vi "SW_Set_Adv_Stimulus_interface.vi"(0 "Zone-based stimulus presents":T1(array[cluster])=[{"Event type"=0, "Time, s"=0.0, "Stimulus, s"=0.0, "Set/Clear"=FALSE, "TTL out"=1, "Stim. has been set"=FALSE}, {"Event type"=0, "Time, s"=0.0, "Stimulus, s"=0.0, "Set/Clear"=FALSE, "TTL out"=1, "Stim. has been set"=FALSE}, {"Event type"=0, "Time, s"=0.0, "Stimulus, s"=0.0, "Set/Clear"=FALSE, "TTL out"=1, "Stim. has been set"=FALSE}, {"Event type"=0, "Time, s"=0.0, "Stimulus, s"=0.0, "Set/Clear"=FALSE, "TTL out"=1, "Stim. has been set"=FALSE}, {"Event type"=0, "Time, s"=0.0, "Stimulus, s"=0.0, "Set/Clear"=FALSE, "TTL out"=1, "Stim. has been set"=FALSE}, {"Event type"=0, "Time, s"=0.0, "Stimulus, s"=0.0, "Set/Clear"=FALSE, "TTL out"=1, "Stim. has been set"=FALSE}, {"Event type"=0, "Time, s"=0.0, "Stimulus, s"=0.0, "Set/Clear"=FALSE, "TTL out"=1, "Stim. has been set"=FALSE}, {"Event type"=0, "Time, s"=0.0, "Stimulus, s"=0.0, "Set/Clear"=FALSE, "TTL out"=1, "Stim. has been set"=FALSE}, {"Event type"=0, "Time, s"=0.0, "Stimulus, s"=0.0, "Set/Clear"=FALSE, "TTL out"=1, "Stim. has been set"=FALSE}, {"Event type"=0, "Time, s"=3.0, "Stimulus, s"=0.3, "Set/Clear"=TRUE, "TTL out"=3, "Stim. has been set"=TRUE}, {"Event type"=0, "Time, s"=0.0, "Stimulus, s"=0.0, "Set/Clear"=FALSE, "TTL out"=1, "Stim. has been set"=FALSE}, {"Event type"=0, "Time, s"=5.0, "Stimulus, s"=1.0, "Set/Clear"=TRUE, "TTL out"=1, "Stim. has been set"=TRUE}, {"Event type"=0, "Time, s"=2.0, "Stimulus, s"=1.0, "Set/Clear"=TRUE, "TTL out"=2, "Stim. has been set"=TRUE}, {"Event type"=0, "Time, s"=0.0, "Stimulus, s"=0.0, "Set/Clear"=FALSE, "TTL out"=1, "Stim. has been set"=FALSE}] {"Event type" items=["Time spent in zone", "Future options"]; "TTL out" items=["1"=1, "2"=2, "1 + 2"=3]}, 1 "Total amount of segments":u32=7, 7 "Run time, s":dbl, 9 "Run time stim, s":dbl, 11 "Run time pause, s":dbl, 12 "Run time threshold, s":dbl, 13 "Speed detection threshold, mm/s":dbl=8.0) -> (3 "Modified Zone-based stimulus presents":T1(array[cluster])=[{"Event type"=0, "Time, s"=0.0, "Stimulus, s"=0.0, "Set/Clear"=FALSE, "TTL out"=1, "Stim. has been set"=FALSE}, {"Event type"=0, "Time, s"=0.0, "Stimulus, s"=0.0, "Set/Clear"=FALSE, "TTL out"=1, "Stim. has been set"=FALSE}, {"Event type"=0, "Time, s"=0.0, "Stimulus, s"=0.0, "Set/Clear"=FALSE, "TTL out"=1, "Stim. has been set"=FALSE}, {"Event type"=0, "Time, s"=0.0, "Stimulus, s"=0.0, "Set/Clear"=FALSE, "TTL out"=1, "Stim. has been set"=FALSE}, {"Event type"=0, "Time, s"=0.0, "Stimulus, s"=0.0, "Set/Clear"=FALSE, "TTL out"=1, "Stim. has been set"=FALSE}, {"Event type"=0, "Time, s"=0.0, "Stimulus, s"=0.0, "Set/Clear"=FALSE, "TTL out"=1, "Stim. has been set"=FALSE}, {"Event type"=0, "Time, s"=0.0, "Stimulus, s"=0.0, "Set/Clear"=FALSE, "TTL out"=1, "Stim. has been set"=FALSE}, {"Event type"=0, "Time, s"=0.0, "Stimulus, s"=0.0, "Set/Clear"=FALSE, "TTL out"=1, "Stim. has been set"=FALSE}, {"Event type"=0, "Time, s"=0.0, "Stimulus, s"=0.0, "Set/Clear"=FALSE, "TTL out"=1, "Stim. has been set"=FALSE}, {"Event type"=0, "Time, s"=3.0, "Stimulus, s"=0.3, "Set/Clear"=TRUE, "TTL out"=3, "Stim. has been set"=TRUE}, {"Event type"=0, "Time, s"=0.0, "Stimulus, s"=0.0, "Set/Clear"=FALSE, "TTL out"=1, "Stim. has been set"=FALSE}, {"Event type"=0, "Time, s"=5.0, "Stimulus, s"=1.0, "Set/Clear"=TRUE, "TTL out"=1, "Stim. has been set"=TRUE}, {"Event type"=0, "Time, s"=2.0, "Stimulus, s"=1.0, "Set/Clear"=TRUE, "TTL out"=2, "Stim. has been set"=TRUE}, {"Event type"=0, "Time, s"=0.0, "Stimulus, s"=0.0, "Set/Clear"=FALSE, "TTL out"=1, "Stim. has been set"=FALSE}] {"Event type" items=["Time spent in zone", "Future options"]; "TTL out" items=["1"=1, "2"=2, "1 + 2"=3]}, 4 "Out Run time, s":dbl, 6 "Out Run time stim, s":dbl, 8 "Out Run time pause, s":dbl, 10 "Out Run time threshold, s":dbl, 15 "Out Speed detection threshold, mm/s":dbl)   [LabVIEW 2016]
uses:
  <vilib>/Utility/miscctls.llb/LVPositionTypeDef.ctl
panel:
  in  "Parameter 5A":dbl=50.0 caption="Speed thresh., mm/s" min=0.0 max=1000.0 step=0.25 format="%.2g"
  out "NewVal":T1(array[cluster])
  out "OldVal":T1(array[cluster])
  in  "Update Zones":bool=TRUE
  in  "Parameter 4A":dbl=50.0 caption="Run time thr., s" min=0.0 max=1000.0 step=0.25 format="%.2g"
  in  "Parameter 3B":dbl=50.0 caption="Time, s" min=0.0 max=1000.0 step=0.25 format="%.2g"
  in  "Parameter 1B":u16(ring) caption="Zone #" items=["Zone 01", "Zone 02", "Zone 03", "Zone 04", "Zone 05", "Zone 06", "Zone 07", "Zone 08", "Zone 09", "Zone 10", "Zone 11", "Zone 12"]
  in  "Parameter 2B":u16(ring) caption="Event type" items=["Time spent in zone", "Future options"]
  in  "Parameter 5B":u16(ring) caption="TTL out" items=["1"=1, "2"=2, "1 + 2"=3]
  out "Navigate Tree:Get Path":string[](array[string])
  in  "Remove Button":bool=TRUE
  in  "Add Button":bool=TRUE
  in  "Modify Button":bool=TRUE
  in  "Reset settings":bool
  in  "Exit":bool
  in  "Save Settings":bool
  in  "Parameter 4B":dbl=50.0 caption="Stimulus, s" min=0.0 max=1000.0 step=0.25 format="%.2g"
  in  "Parameter 3A":dbl=50.0 caption="Stimulus, s" min=0.0 max=1000.0 step=0.25 format="%.2g"
  in  "Parameter 2A":dbl=50.0 caption="Pause, s" min=0.0 max=1000.0 step=0.25 format="%.2f"
  in  "Parameter 1A":dbl=50.0 caption="Runnig, s" min=0.0 max=1000.0 step=0.25 format="%.2g"
  in  "TTL firing conditions":string(tree)
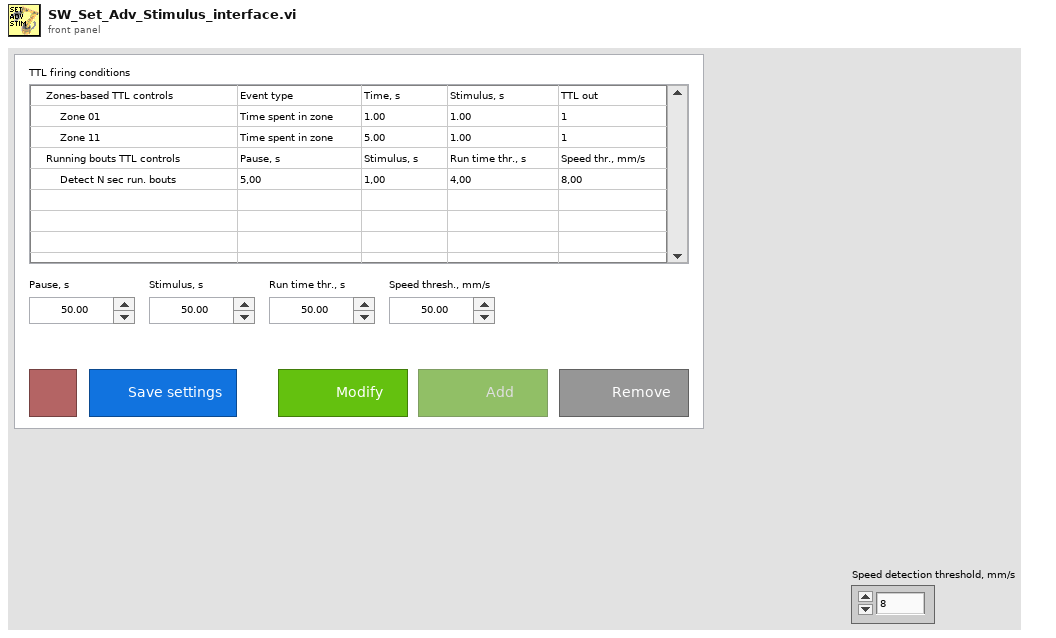
[diagram p1: front panel]
types:
  T1 = cluster{"Event type":u16, "Time, s":sgl, "Stimulus, s":sgl, "Set/Clear":bool, "TTL out":u16, "Stim. has been set":bool}[]
  T2 = typedef "LVPositionTypeDef.ctl" = cluster{"Left":i32, "Top":i32}
  T3 = typedef "LVStringsAndValuesArrayTypeDef_U16.ctl" = cluster{"String":string, "Value":u16}[]
  T4 = enum8{"Enabled", "Disabled", "Disabled and Grayed Out"}
  T5 = cluster{"Event type":u16, "Time, s":sgl, "Stimulus, s":sgl, "Set/Clear":bool, "TTL out":u16, "Stim. has been set":bool}
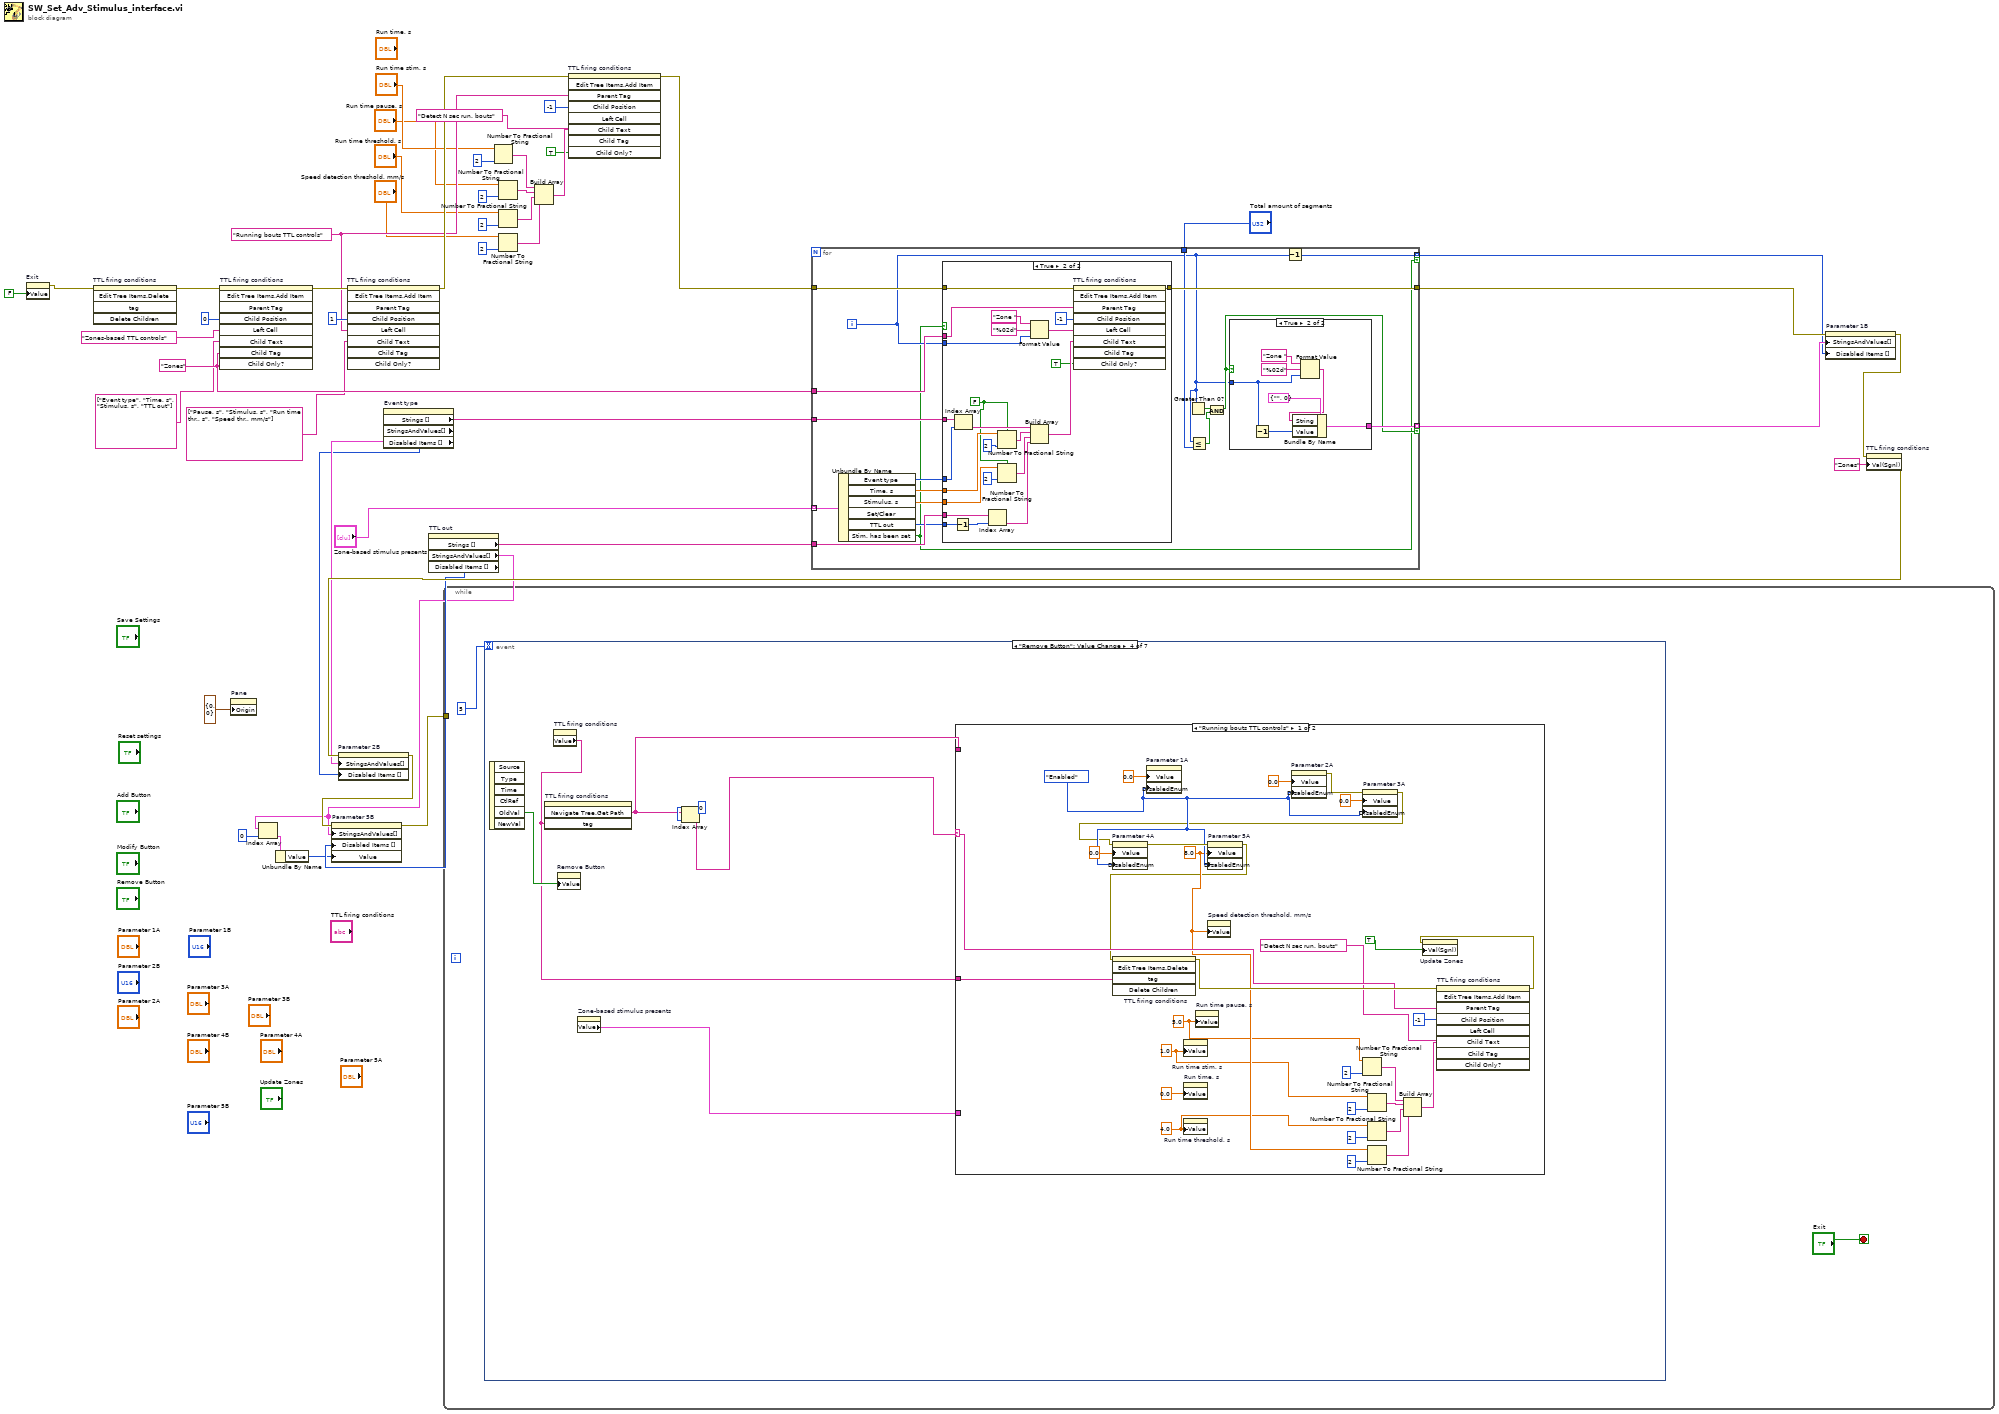
[diagram p0: block diagram]
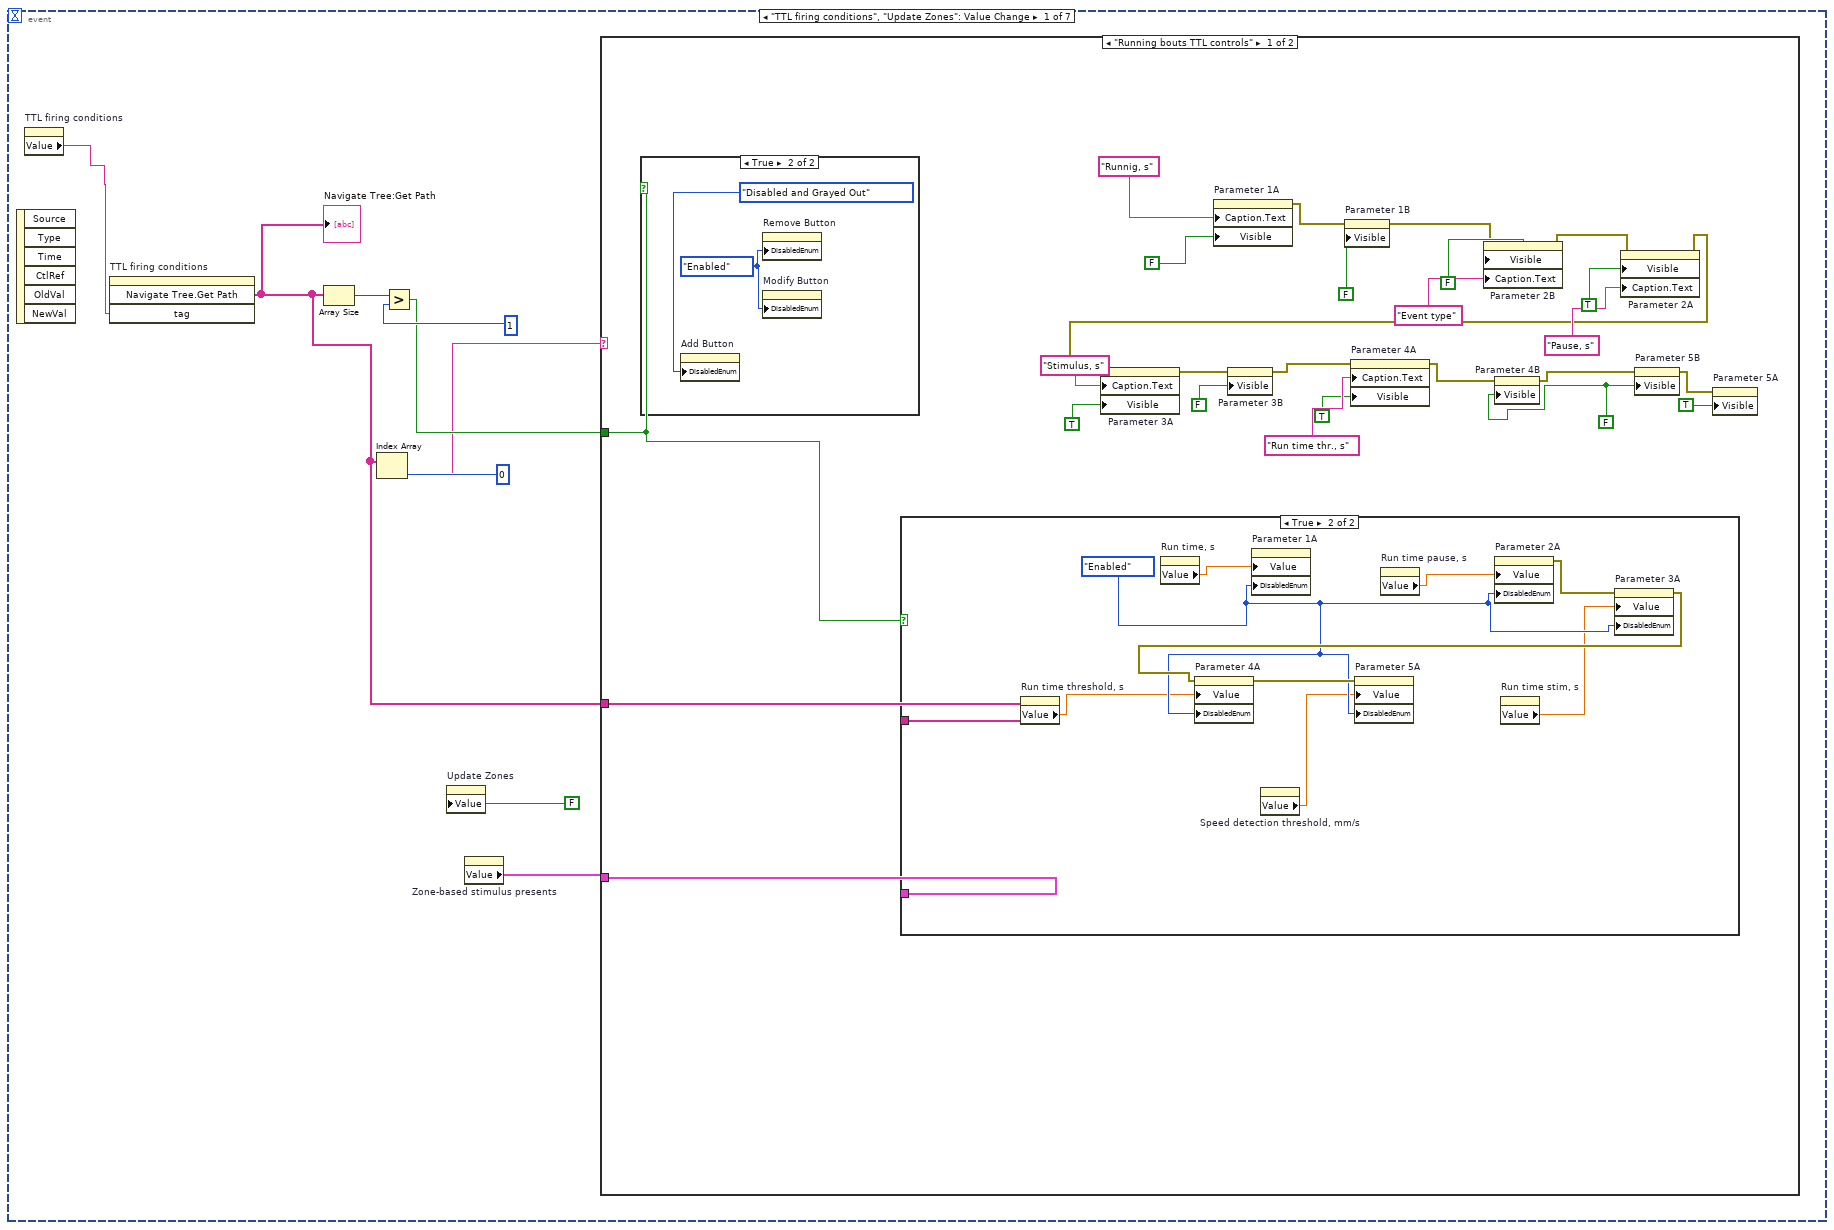
[diagram p2: hidden frame]
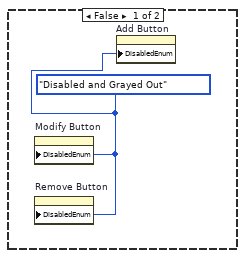
[diagram p3: hidden frame]
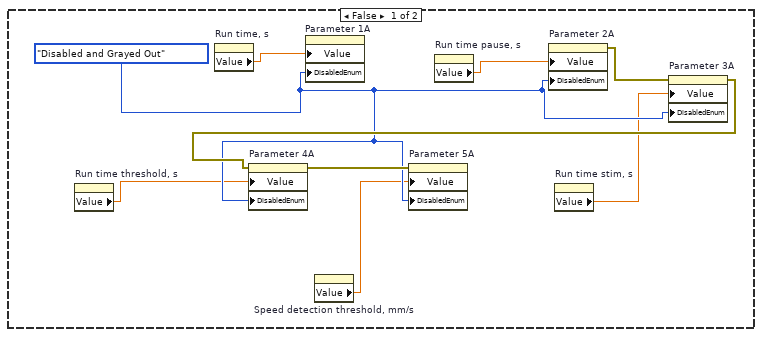
[diagram p4: hidden frame]
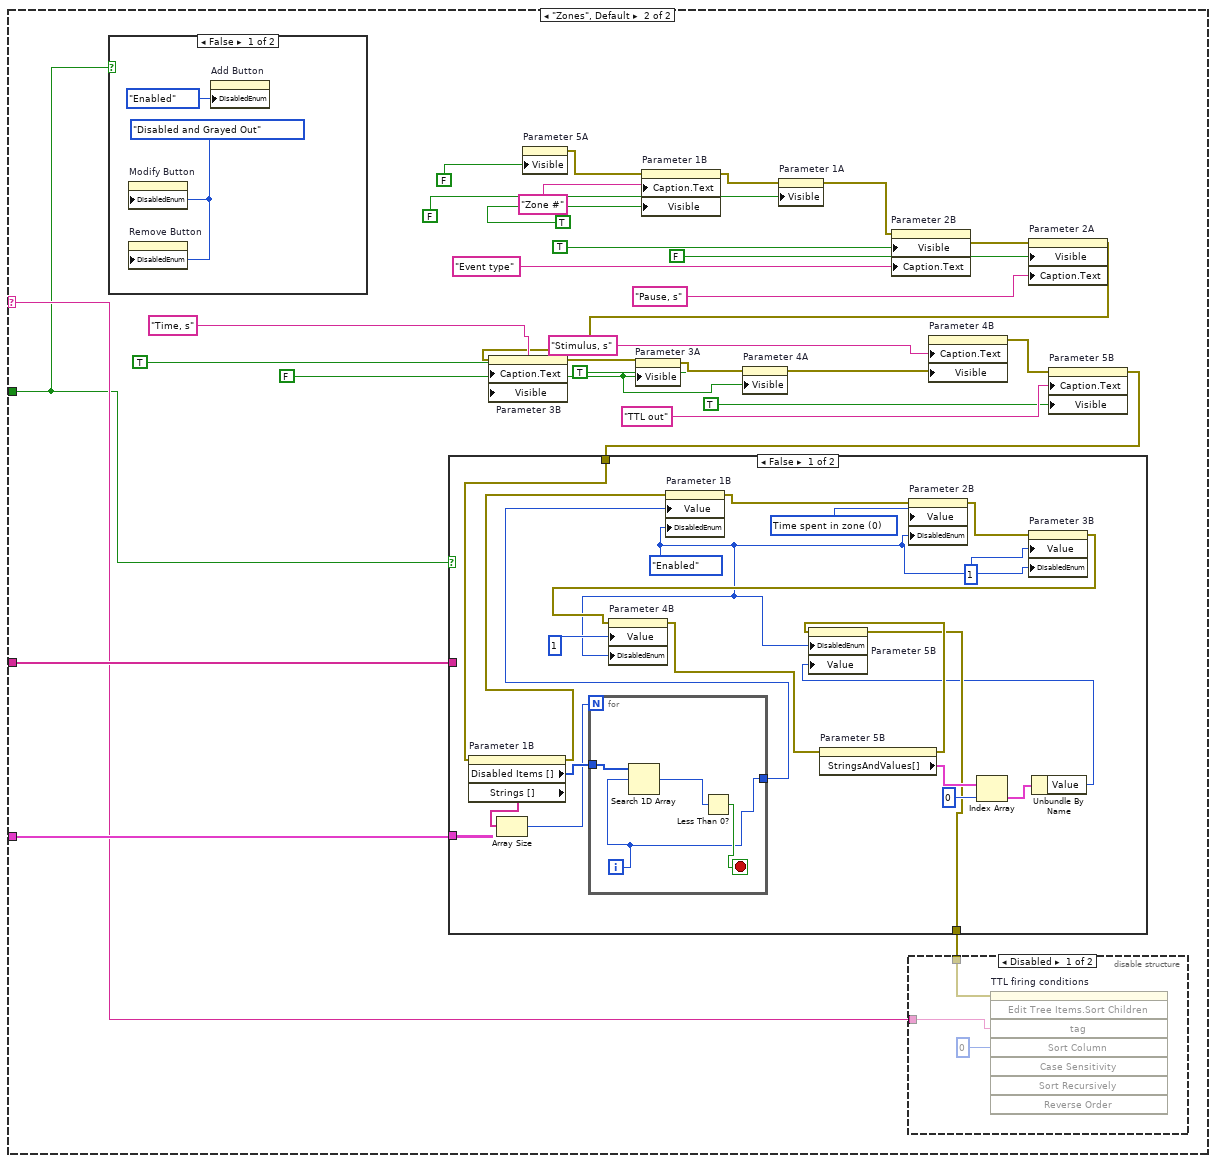
[diagram p5: hidden frame]
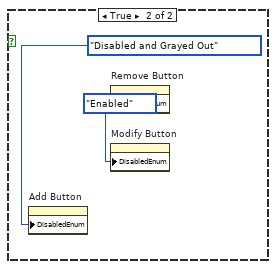
[diagram p6: hidden frame]
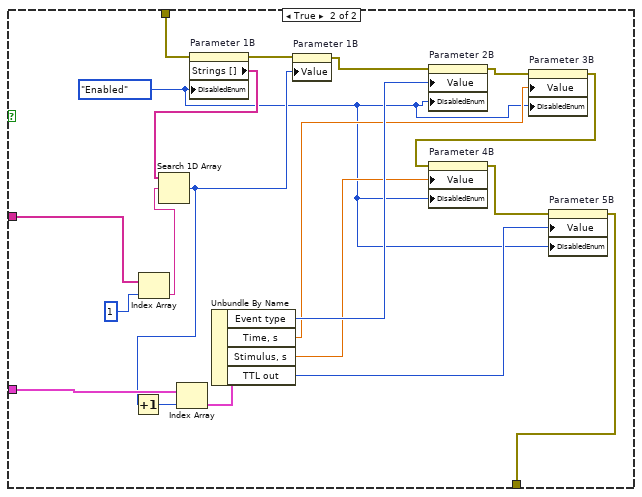
[diagram p8: hidden frame]
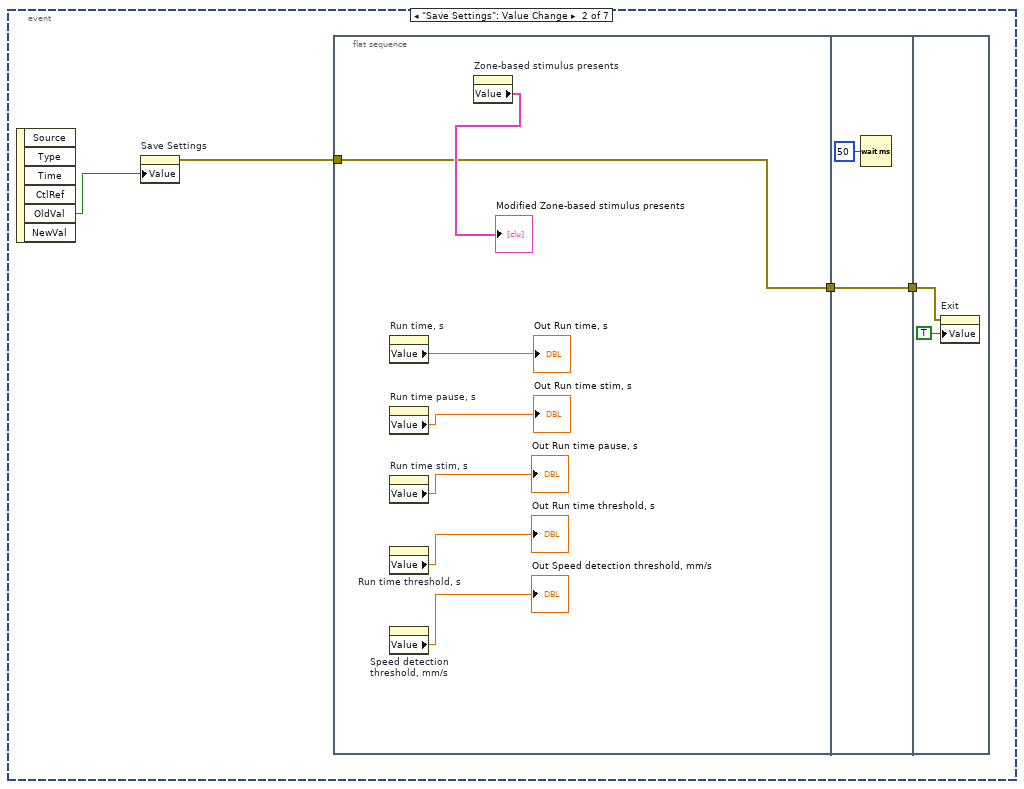
[diagram p9: hidden frame]
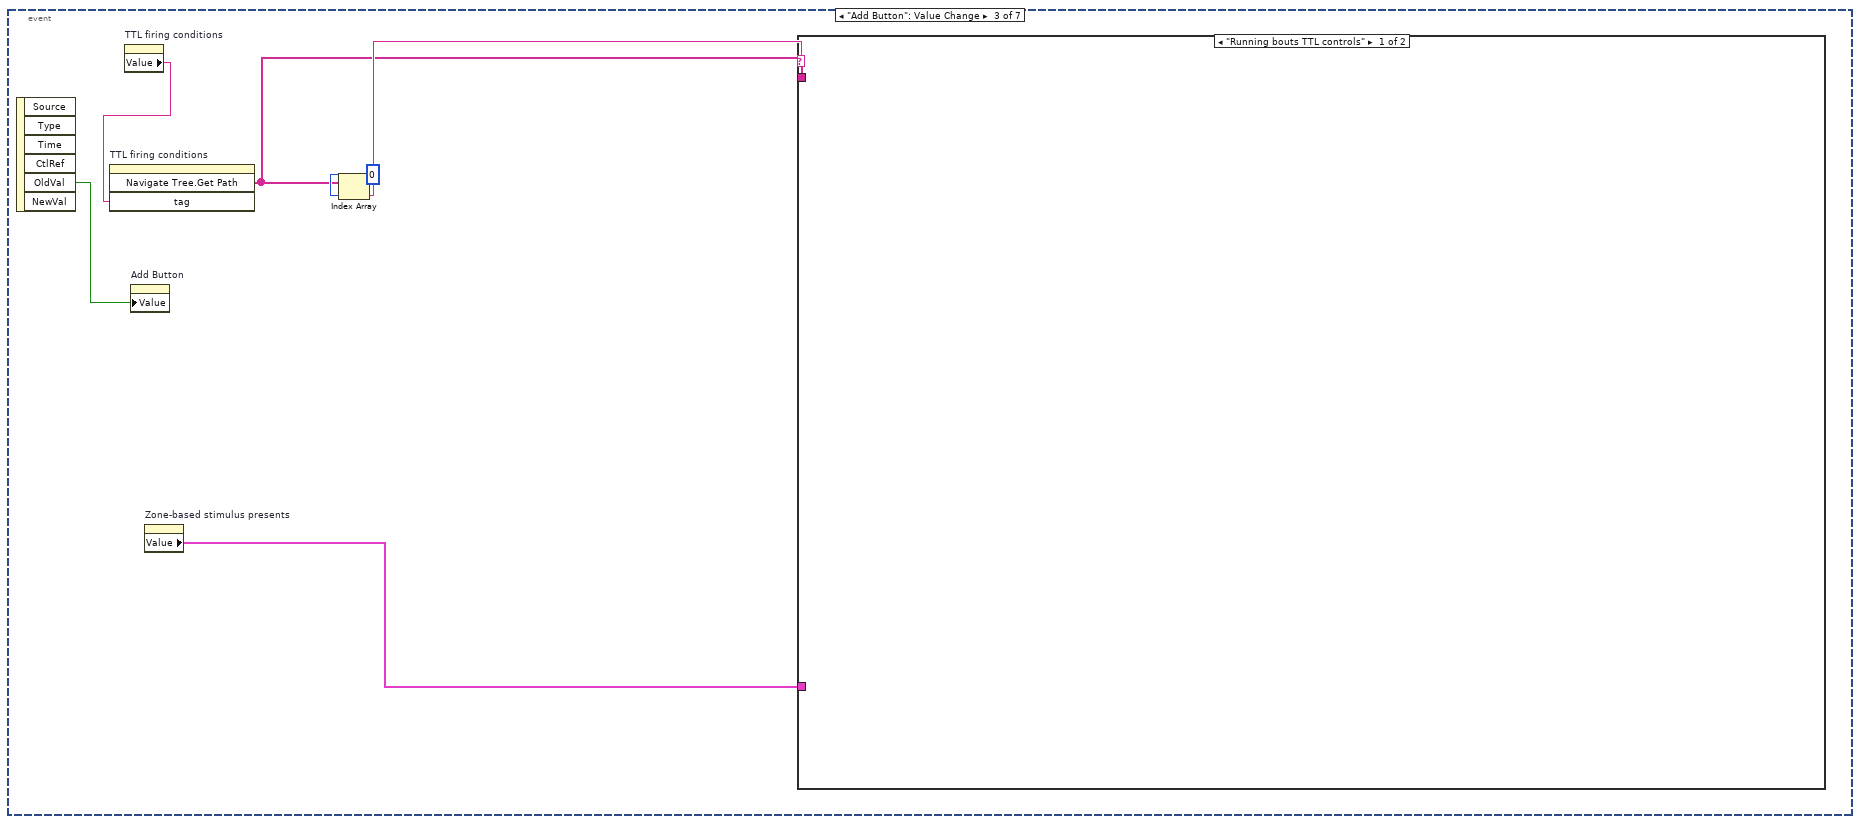
[diagram p10: hidden frame]
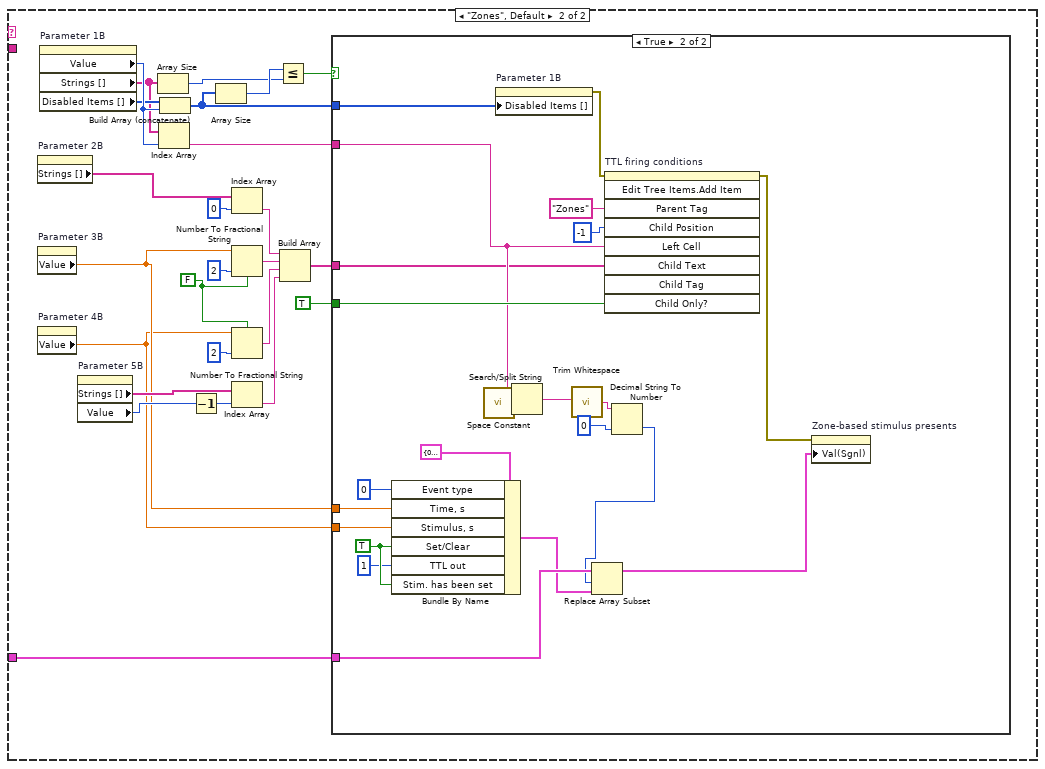
[diagram p11: hidden frame]
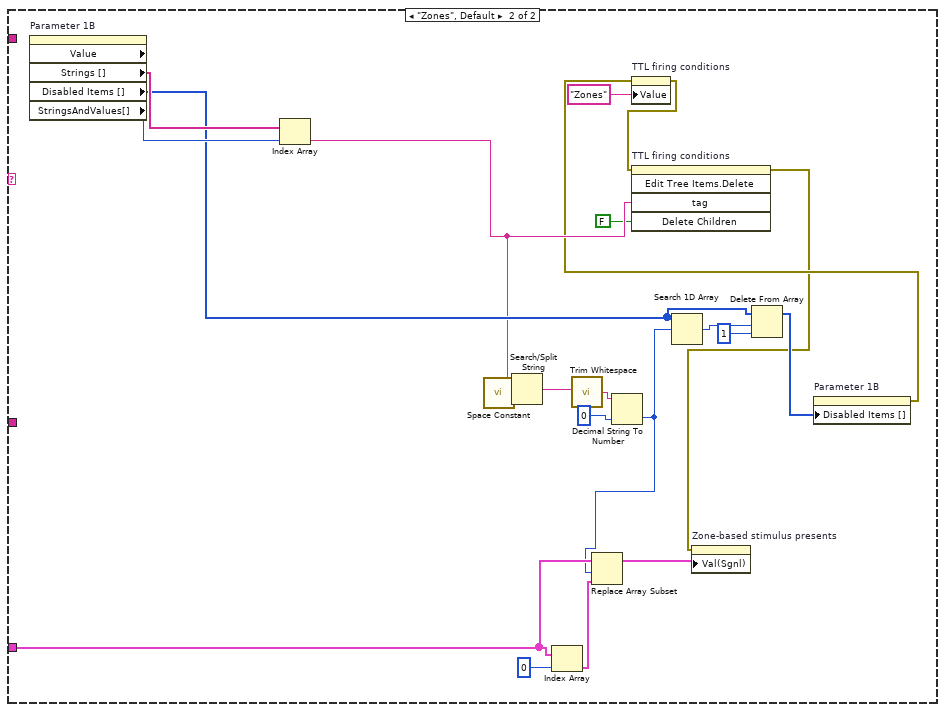
[diagram p13: hidden frame]
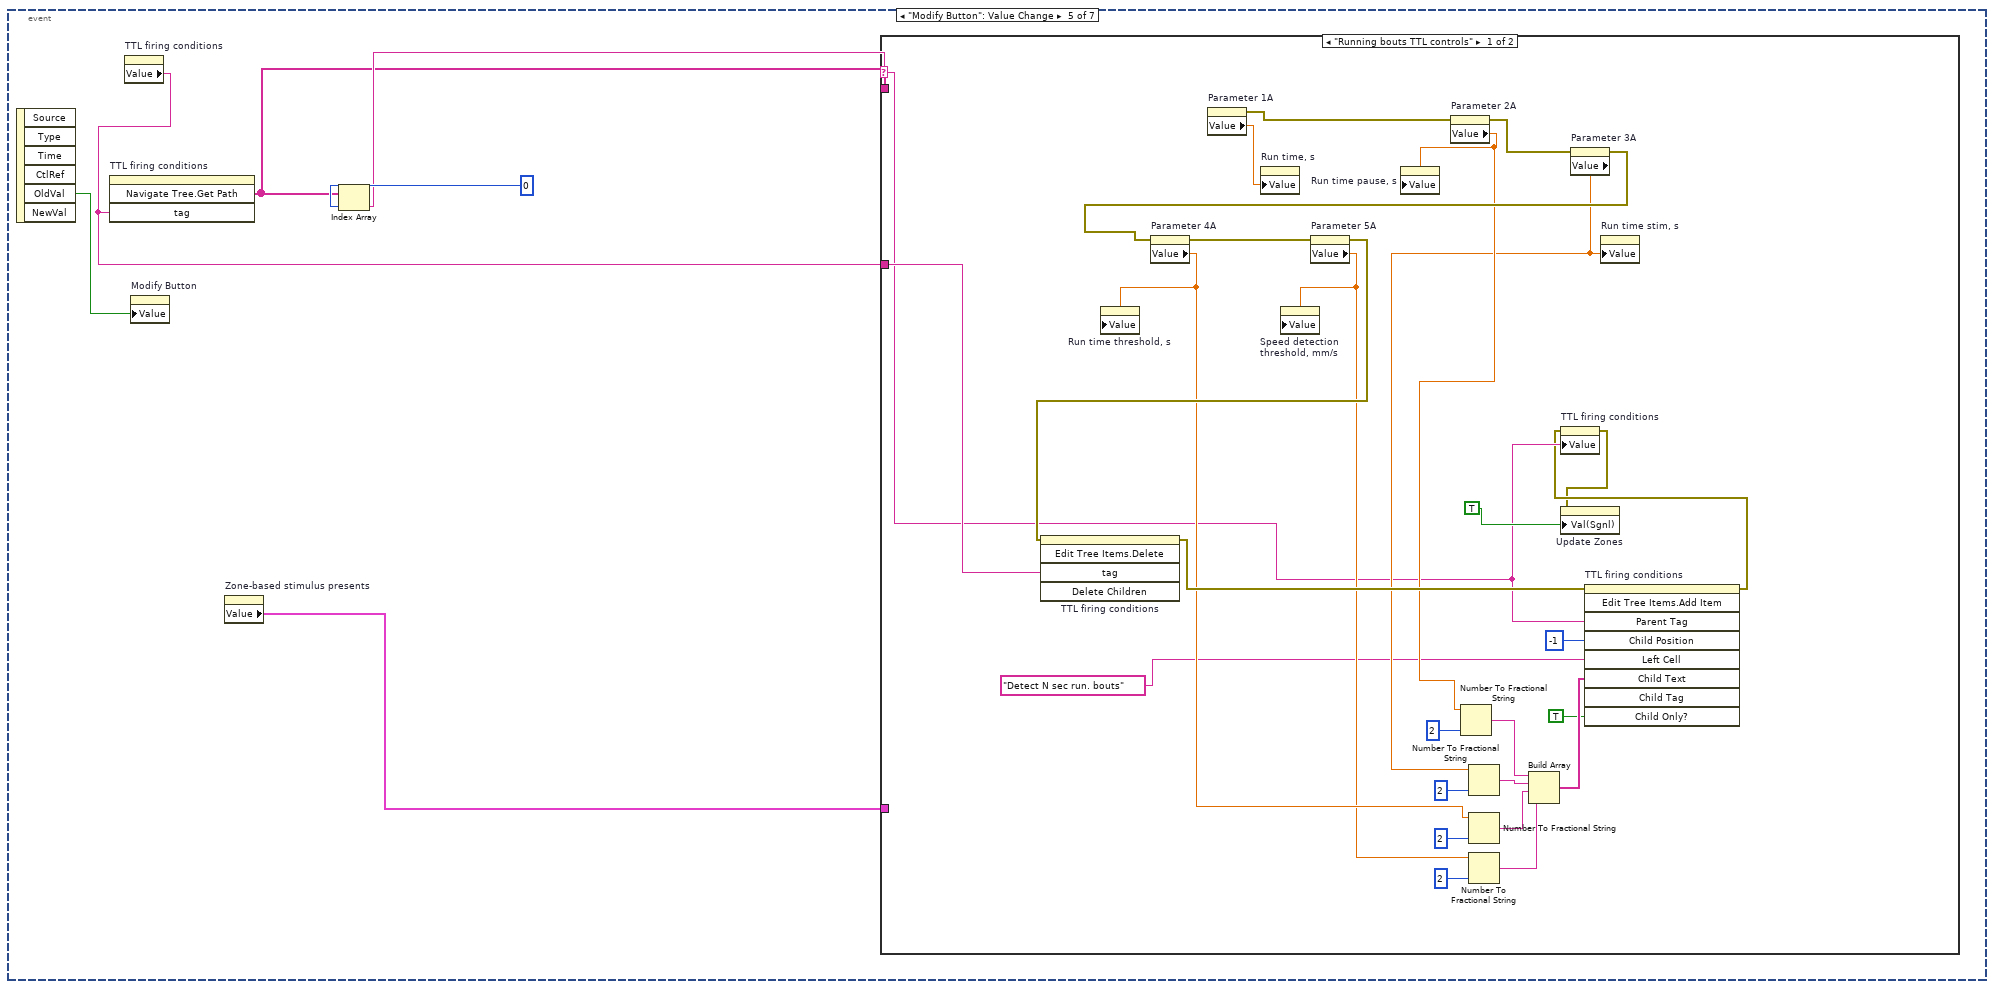
[diagram p14: hidden frame]
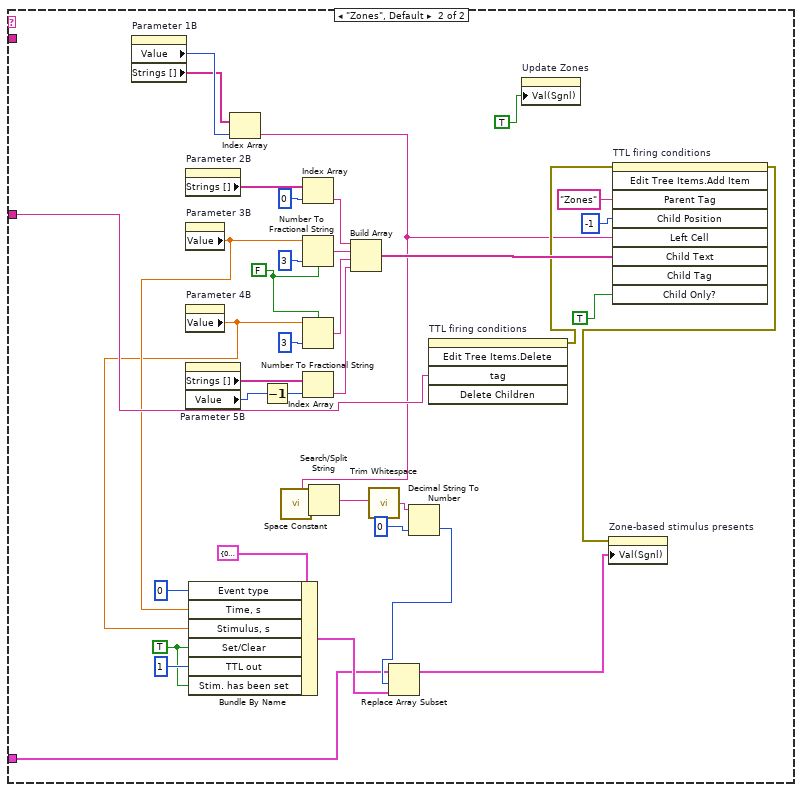
[diagram p15: hidden frame]
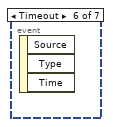
[diagram p16: hidden frame]
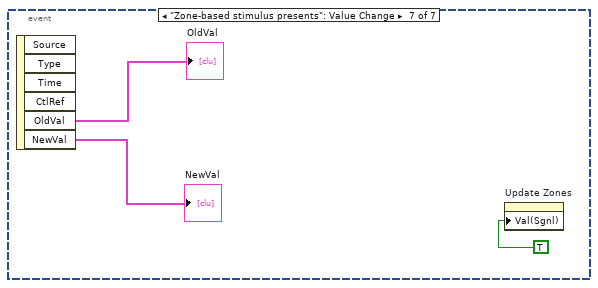
[diagram p17: hidden frame]
diagram:
  w19 = "Running bouts TTL controls" ("Parent Tag")
  w47 = "Zones" ("Child Tag")
  n1 = property on="Exit" class="Bool (strict)"("Value"=FALSE ("Exit")) -> (error out=w3:errorcluster)  [unwired: 2 in, 1 out]
  n2 = invoke on="TTL firing conditions" class="Tree (strict)" method="Edit Tree Items.Delete"(error in=w3) -> (error out=w48:errorcluster)  [unwired: 4 in, 4 out]
  n3 = invoke on="TTL firing conditions" class="Tree (strict)" method="Edit Tree Items.Add Item"(error in=w48, "Child Position"=0, "Left Cell"="Zones-based TTL controls" ("Parent Tag"), "Child Text"=string[] ["Event type", "Time, s", "Stimulus, s", "TTL out"], "Child Tag"=w47) -> (error out=w44:errorcluster)  [unwired: 4 in, 8 out]
  n4 = property on="Pane" class="Pane"("Origin"=T2 {"Left"=0, "Top"=0} ("Position")) -> ()  [unwired: 2 in, 2 out]
  n5 = invoke on="TTL firing conditions" class="Tree (strict)" method="Edit Tree Items.Add Item"(error in=w44, "Child Position"=1, "Left Cell"=w19, "Child Text"=string[] ["Pause, s", "Stimulus, s", "Run time thr., s", "Speed thr., mm/s"]) -> (error out=w21:errorcluster)  [unwired: 5 in, 8 out]
  n6 = property on="Event type" class="Ring (strict)"() -> ("Strings []"=w37:string[], "StringsAndValues[]"=w36:T3, "Disabled Items []"=w35:i32[])  [unwired: 2 in, 2 out]
  n7 = property on="TTL out" class="Ring (strict)"() -> ("Strings []"=w45:string[], "StringsAndValues[]"=w31:T3, "Disabled Items []"=w32:i32[])  [unwired: 2 in, 2 out]
  n8 = Index Array(array=w31, index=0) -> (element=w29:cluster{"String":string, "Value":u16})
  n9 = Unbundle By Name(w29) -> ("Value"=w28:u16)
  n10 = Number To Fractional String(number="Run time stim, s", precision (6)=i16 2) -> (F-format string=w9:string)  [unwired: 2 in]
  n11 = Number To Fractional String(number="Run time pause, s", precision (6)=i16 2) -> (F-format string=w8:string)  [unwired: 2 in]
  n12 = Number To Fractional String(number="Run time threshold, s", precision (6)=i16 2) -> (F-format string=w7:string)  [unwired: 2 in]
  n13 = Number To Fractional String(number="Speed detection threshold, mm/s", precision (6)=i16 2) -> (F-format string=w6:string)  [unwired: 2 in]
  n14 = Build Array(w9, w8, w7, w6) -> (w5:string[])
  n15 = invoke on="TTL firing conditions" class="Tree (strict)" method="Edit Tree Items.Add Item"(error in=w21, "Parent Tag"=w19, "Child Position"=-1, "Left Cell"="Detect N sec run. bouts" ("Left Cell String"), "Child Text"=w5, "Child Only?"=TRUE) -> (error out=w20:errorcluster)  [unwired: 3 in, 8 out]
  n16 = for {
    tunnel: "Zone-based stimulus presents" -> [w67] mode=indexing
    tunnel: w20 -> [w66]
    tunnel: w47 -> [w65]
    tunnel: w37 -> [w63]
    tunnel: w45 -> [w60]
    tunnel: [w58] -> w27
    tunnel: [w57] -> w26 mode=indexing if=w55
    tunnel: "Total amount of segments" -> [w56]
    tunnel: [w50] -> w24 mode=indexing if=w51
    i -> [w52]
    n17 = Unbundle By Name(w67) -> ("Event type"=w62:u16, "Time, s"=w64:sgl, "Stimulus, s"=w61:sgl, "TTL out"=w59:u16, "Stim. has been set"=w51:bool)  [unwired: 1 out]
    n18 = case shown="True" w51 {
      tunnel: w66 -> [_ w98]
      tunnel: w65 -> [_ w97]
      tunnel: w52 -> [_ w91]
      tunnel: w64 -> [_ w92]
      tunnel: w63 -> [_ w90]
      tunnel: w62 -> [_ w86]
      tunnel: w61 -> [_ w85]
      tunnel: w60 -> [_ w81]
      tunnel: w59 -> [_ w80]
      tunnel: [_ w76] -> w58
      frame False {
      }
      frame True {
        w75 = FALSE ("use system decimal point (T)")
        n19 = Decrement(x=w80) -> (x-1=w78:u16)
        n20 = Index Array(array=w90, index=w86) -> (element=w89:string)
        n21 = Index Array(array=w81, index=w78) -> (element=w79:string)
        n22 = Number To Fractional String(use system decimal point (T)=w75, number=w92, precision (6)=i16 2) -> (F-format string=w88:string)  [unwired: 1 in]
        n23 = Number To Fractional String(use system decimal point (T)=w75, number=w85, precision (6)=i16 2) -> (F-format string=w84:string)  [unwired: 1 in]
        n24 = Format Value(string ("")="Zone " ("string"), format string="%02d", value (0)=w91) -> (output string=w94:string)
        n25 = Build Array(w89, w88, w84, w79) -> (w87:string[])
        n26 = invoke on="TTL firing conditions" class="Tree (strict)" method="Edit Tree Items.Add Item"(error in=w98, "Parent Tag"=w97, "Child Position"=-1, "Left Cell"=w94, "Child Text"=w87, "Child Only?"=TRUE) -> (error out=w76:errorcluster)  [unwired: 3 in, 8 out]
      }
    }
    n27 = Greater Than 0?(x=w52) -> (x > 0?=w54:bool)
    n28 = Less Or Equal?(x=w52, y=w56) -> (x <= y?=w53:bool)
    n29 = And(x=w54, y=w53) -> (x .and. y?=w55:bool)
    n30 = case shown="True" w55 {
      tunnel: w52 -> [_ w71]
      tunnel: [_ w68] -> w57
      frame False {
      }
      frame True {
        n31 = Decrement(x=w71) -> (x-1=w70:i32)
        n32 = Format Value(string ("")="Zone " ("string"), format string="%02d", value (0)=w71) -> (output string=w69:string)
        n33 = Bundle By Name(cluster=cluster{"String":string, "Value":u16} {"String"="", "Value"=0} ("Zones available for selection"), "String"=w69, "Value"=w70) -> (w68:cluster{"String":string, "Value":u16})
      }
    }
    n34 = Decrement(x=w52) -> (x-1=w50:i32)
  }
  n35 = property on="Parameter 1B" class="Ring (strict)"(error in=w27, "StringsAndValues[]"=w26, "Disabled Items []"=w24) -> (error out=w23:errorcluster)  [unwired: 1 in, 1 out]
  n36 = property on="TTL firing conditions" class="Tree (strict)"(error in=w23, "Val(Sgnl)"="Zones" ("TTL firing conditions")) -> (error out=w38:errorcluster)  [unwired: 1 in, 1 out]
  n37 = property on="Parameter 2B" class="Ring (strict)"(error in=w38, "StringsAndValues[]"=w36, "Disabled Items []"=w35) -> (error out=w34:errorcluster)  [unwired: 1 in, 1 out]
  n38 = property on="Parameter 5B" class="Ring (strict)"(error in=w34, "StringsAndValues[]"=w31, "Disabled Items []"=w32, "Value"=w28) -> (error out=w33:errorcluster)  [unwired: 1 in, 1 out]
  n39 = while {
    tunnel: w33 -> [w100]
    tunnel: [w100] -> _
    stop <- "Exit" stop-if-true
    n40 = event shown="[3] \"Remove Button\": Value Change" {
      selector: _ -> [_ _ _ _ _ _ _]
      dyn-events: _ -> [_ _ _ _ _ _ _]
      timeout: 5 -> [_ _ _ _ _ _ _]
      event "TTL firing conditions", "Update Zones": Value Change {
        n41 = event-data() -> ()  [unwired: 1 in, 6 out]
        n42 = property on="TTL firing conditions" class="Tree (strict)"() -> ("Value"=w103:string)  [unwired: 2 in, 2 out]
        n43 = invoke on="TTL firing conditions" class="Tree (strict)" method="Navigate Tree.Get Path"("tag"=w103) -> ("Navigate Tree:Get Path"=w105:string[])  [unwired: 3 in, 3 out]
        "Navigate Tree:Get Path" <- w105
        n44 = Array Size(array=w105) -> (size(s)=w110:i32)
        n45 = Index Array(array=w105, index=0) -> (element=w106:string)
        n46 = Greater?(x=w110, y=1) -> (0:w107:bool)
        n47 = property on="Update Zones" class="Bool (strict)"("Value"=FALSE ("Update Zones")) -> ()  [unwired: 2 in, 2 out]
        n48 = property on="Zone-based stimulus presents" class="Arr (strict)"() -> ("Value"=w102:T1)  [unwired: 2 in, 2 out]
        n49 = case shown="\"Running bouts TTL controls\"" w106 {
          selector: w106 -> [_ w161]
          tunnel: w107 -> [w111 w158]
          tunnel: w105 -> [w122 w173]
          tunnel: w102 -> [w123 w172]
          frame "Running bouts TTL controls" {
            w114 = FALSE ("Visible")
            n50 = case shown="True" w111 {
              frame False {
                w137 = T4."Disabled and Grayed Out" ("Disabled")
                n51 = property on="Modify Button" class="Bool (strict)"("DisabledEnum"=w137) -> ()  [unwired: 2 in, 2 out]
                n52 = property on="Remove Button" class="Bool (strict)"("DisabledEnum"=w137) -> ()  [unwired: 2 in, 2 out]
                n53 = property on="Add Button" class="Bool (strict)"("DisabledEnum"=w137) -> ()  [unwired: 2 in, 2 out]
              }
              frame True {
                w138 = T4."Enabled" ("Disabled")
                n54 = property on="Add Button" class="Bool (strict)"("DisabledEnum"=T4."Disabled and Grayed Out" ("Disabled")) -> ()  [unwired: 2 in, 2 out]
                n55 = property on="Remove Button" class="Bool (strict)"("DisabledEnum"=w138) -> ()  [unwired: 2 in, 2 out]
                n56 = property on="Modify Button" class="Bool (strict)"("DisabledEnum"=w138) -> ()  [unwired: 2 in, 2 out]
              }
            }
            n57 = case shown="True" w111 {
              tunnel: w122 -> [_ _]
              tunnel: w123 -> [_ _]
              frame False {
                w145 = T4."Disabled and Grayed Out" ("Disabled")
                n58 = property on="Run time threshold, s" class="DigNum (strict)"() -> ("Value"=w141:dbl)  [unwired: 2 in, 2 out]
                n59 = property on="Run time, s" class="DigNum (strict)"() -> ("Value"=w144:dbl)  [unwired: 2 in, 2 out]
                n60 = property on="Parameter 1A" class="DigNum (strict)"("Value"=w144, "DisabledEnum"=w145) -> ()  [unwired: 2 in, 2 out]
                n61 = property on="Speed detection threshold, mm/s" class="DigNum (strict)"() -> ("Value"=w140:dbl)  [unwired: 2 in, 2 out]
                n62 = property on="Run time pause, s" class="DigNum (strict)"() -> ("Value"=w143:dbl)  [unwired: 2 in, 2 out]
                n63 = property on="Parameter 2A" class="DigNum (strict)"("Value"=w143, "DisabledEnum"=w145) -> (error out=w148:errorcluster)  [unwired: 2 in, 1 out]
                n64 = property on="Run time stim, s" class="DigNum (strict)"() -> ("Value"=w142:dbl)  [unwired: 2 in, 2 out]
                n65 = property on="Parameter 3A" class="DigNum (strict)"(error in=w148, "Value"=w142, "DisabledEnum"=w145) -> (error out=w146:errorcluster)  [unwired: 1 in, 1 out]
                n66 = property on="Parameter 4A" class="DigNum (strict)"(error in=w146, "Value"=w141, "DisabledEnum"=w145) -> (error out=w147:errorcluster)  [unwired: 1 in, 1 out]
                n67 = property on="Parameter 5A" class="DigNum (strict)"(error in=w147, "Value"=w140, "DisabledEnum"=w145) -> ()  [unwired: 1 in, 2 out]
              }
              frame True {
                w154 = T4."Enabled" ("Disabled")
                n68 = property on="Run time threshold, s" class="DigNum (strict)"() -> ("Value"=w150:dbl)  [unwired: 2 in, 2 out]
                n69 = property on="Run time, s" class="DigNum (strict)"() -> ("Value"=w153:dbl)  [unwired: 2 in, 2 out]
                n70 = property on="Parameter 1A" class="DigNum (strict)"("Value"=w153, "DisabledEnum"=w154) -> ()  [unwired: 2 in, 2 out]
                n71 = property on="Speed detection threshold, mm/s" class="DigNum (strict)"() -> ("Value"=w149:dbl)  [unwired: 2 in, 2 out]
                n72 = property on="Run time pause, s" class="DigNum (strict)"() -> ("Value"=w152:dbl)  [unwired: 2 in, 2 out]
                n73 = property on="Parameter 2A" class="DigNum (strict)"("Value"=w152, "DisabledEnum"=w154) -> (error out=w157:errorcluster)  [unwired: 2 in, 1 out]
                n74 = property on="Run time stim, s" class="DigNum (strict)"() -> ("Value"=w151:dbl)  [unwired: 2 in, 2 out]
                n75 = property on="Parameter 3A" class="DigNum (strict)"(error in=w157, "Value"=w151, "DisabledEnum"=w154) -> (error out=w155:errorcluster)  [unwired: 1 in, 1 out]
                n76 = property on="Parameter 4A" class="DigNum (strict)"(error in=w155, "Value"=w150, "DisabledEnum"=w154) -> (error out=w156:errorcluster)  [unwired: 1 in, 1 out]
                n77 = property on="Parameter 5A" class="DigNum (strict)"(error in=w156, "Value"=w149, "DisabledEnum"=w154) -> ()  [unwired: 1 in, 2 out]
              }
            }
            n78 = property on="Parameter 1A" class="DigNum (strict)"("Caption.Text"="Runnig, s", "Visible"=FALSE) -> (error out=w133:errorcluster)  [unwired: 2 in, 1 out]
            n79 = property on="Parameter 1B" class="Ring (strict)"(error in=w133, "Visible"=FALSE) -> (error out=w129:errorcluster)  [unwired: 1 in, 1 out]
            n80 = property on="Parameter 2B" class="Ring (strict)"(error in=w129, "Visible"=FALSE, "Caption.Text"="Event type") -> (error out=w131:errorcluster)  [unwired: 1 in, 1 out]
            n81 = property on="Parameter 2A" class="DigNum (strict)"(error in=w131, "Visible"=TRUE, "Caption.Text"="Pause, s") -> (error out=w125:errorcluster)  [unwired: 1 in, 1 out]
            n82 = property on="Parameter 3A" class="DigNum (strict)"(error in=w125, "Caption.Text"="Stimulus, s", "Visible"=TRUE) -> (error out=w120:errorcluster)  [unwired: 1 in, 1 out]
            n83 = property on="Parameter 3B" class="DigNum (strict)"(error in=w120, "Visible"=FALSE) -> (error out=w119:errorcluster)  [unwired: 1 in, 1 out]
            n84 = property on="Parameter 4A" class="DigNum (strict)"(error in=w119, "Caption.Text"="Run time thr., s", "Visible"=TRUE) -> (error out=w116:errorcluster)  [unwired: 1 in, 1 out]
            n85 = property on="Parameter 4B" class="DigNum (strict)"(error in=w116, "Visible"=w114) -> (error out=w115:errorcluster)  [unwired: 1 in, 1 out]
            n86 = property on="Parameter 5B" class="Ring (strict)"(error in=w115, "Visible"=w114) -> (error out=w113:errorcluster)  [unwired: 1 in, 1 out]
            n87 = property on="Parameter 5A" class="DigNum (strict)"(error in=w113, "Visible"=TRUE) -> ()  [unwired: 1 in, 2 out]
          }
          frame "Zones", Default {
            w166 = FALSE ("Visible")
            n88 = case shown="False" w158 {
              frame False {
                w189 = T4."Disabled and Grayed Out" ("Disabled")
                n89 = property on="Modify Button" class="Bool (strict)"("DisabledEnum"=w189) -> ()  [unwired: 2 in, 2 out]
                n90 = property on="Remove Button" class="Bool (strict)"("DisabledEnum"=w189) -> ()  [unwired: 2 in, 2 out]
                n91 = property on="Add Button" class="Bool (strict)"("DisabledEnum"=T4."Enabled" ("Disabled")) -> ()  [unwired: 2 in, 2 out]
              }
              frame True {
                w191 = T4."Enabled" ("Disabled")
                n92 = property on="Add Button" class="Bool (strict)"("DisabledEnum"=T4."Disabled and Grayed Out" ("Disabled")) -> ()  [unwired: 2 in, 2 out]
                n93 = property on="Remove Button" class="Bool (strict)"("DisabledEnum"=w191) -> ()  [unwired: 2 in, 2 out]
                n94 = property on="Modify Button" class="Bool (strict)"("DisabledEnum"=w191) -> ()  [unwired: 2 in, 2 out]
              }
            }
            n95 = property on="Parameter 5A" class="DigNum (strict)"("Visible"=FALSE) -> (error out=w159:errorcluster)  [unwired: 2 in, 1 out]
            n96 = property on="Parameter 1B" class="Ring (strict)"(error in=w159, "Caption.Text"="Zone #" ("Label.Text"), "Visible"=TRUE) -> (error out=w184:errorcluster)  [unwired: 1 in, 1 out]
            n97 = property on="Parameter 1A" class="DigNum (strict)"(error in=w184, "Visible"=FALSE) -> (error out=w178:errorcluster)  [unwired: 1 in, 1 out]
            n98 = property on="Parameter 2B" class="Ring (strict)"(error in=w178, "Visible"=TRUE, "Caption.Text"="Event type") -> (error out=w182:errorcluster)  [unwired: 1 in, 1 out]
            n99 = property on="Parameter 2A" class="DigNum (strict)"(error in=w182, "Visible"=FALSE, "Caption.Text"="Pause, s") -> (error out=w168:errorcluster)  [unwired: 1 in, 1 out]
            n100 = property on="Parameter 3B" class="DigNum (strict)"(error in=w168, "Caption.Text"="Time, s", "Visible"=TRUE) -> (error out=w167:errorcluster)  [unwired: 1 in, 1 out]
            n101 = property on="Parameter 3A" class="DigNum (strict)"(error in=w167, "Visible"=w166) -> (error out=w165:errorcluster)  [unwired: 1 in, 1 out]
            n102 = property on="Parameter 4A" class="DigNum (strict)"(error in=w165, "Visible"=w166) -> (error out=w164:errorcluster)  [unwired: 1 in, 1 out]
            n103 = property on="Parameter 4B" class="DigNum (strict)"(error in=w164, "Caption.Text"="Stimulus, s", "Visible"=TRUE) -> (error out=w176:errorcluster)  [unwired: 1 in, 1 out]
            n104 = property on="Parameter 5B" class="Ring (strict)"(error in=w176, "Caption.Text"="TTL out", "Visible"=TRUE) -> (error out=w171:errorcluster)  [unwired: 1 in, 1 out]
            n105 = case shown="False" w158 {
              tunnel: w173 -> [_ w234]
              tunnel: w172 -> [_ w232]
              tunnel: w171 -> [w199 w221]
              tunnel: [w196 w219] -> w162
              frame False {
                w214 = u16 0 items=["Time spent in zone", "Future options"] ("Parameter 2B")
                w209 = T4."Enabled" ("Disabled")
                n106 = property on="Parameter 1B" class="Ring (strict)"(error in=w199) -> (error out=w206:errorcluster, "Disabled Items []"=w208:i32[], "Strings []"=w204:string[])  [unwired: 1 in, 1 out]
                n107 = Array Size(array=w204) -> (size(s)=w203:i32)
                n108 = for {
                  N: w203 -> [_]
                  tunnel: w208 -> [w218]
                  tunnel: [w215] -> w205
                  i -> [w215]
                  stop <- w217 stop-if-true
                  n109 = Search 1D Array(1D array=w218, element=w215) -> (index of element=w216:i32)  [unwired: 1 in]
                  n110 = Less Than 0?(x=w216) -> (x < 0?=w217:bool)
                }
                n111 = property on="Parameter 1B" class="Ring (strict)"(error in=w206, "Value"=w205, "DisabledEnum"=w209) -> (error out=w207:errorcluster)  [unwired: 1 in, 1 out]
                n112 = property on="Parameter 2B" class="Ring (strict)"(error in=w207, "Value"=w214, "DisabledEnum"=w209) -> (error out=w213:errorcluster)  [unwired: 1 in, 1 out]
                n113 = property on="Parameter 3B" class="DigNum (strict)"(error in=w213, "Value"=u16 1 ("Parameter 3A"), "DisabledEnum"=w209) -> (error out=w210:errorcluster)  [unwired: 1 in, 1 out]
                n114 = property on="Parameter 4B" class="DigNum (strict)"(error in=w210, "Value"=u16 1 ("Parameter 4A"), "DisabledEnum"=w209) -> (error out=w198:errorcluster)  [unwired: 1 in, 1 out]
                n115 = property on="Parameter 5B" class="Ring (strict)"(error in=w198) -> (error out=w197:errorcluster, "StringsAndValues[]"=w202:T3)  [unwired: 1 in, 1 out]
                n116 = Index Array(array=w202, index=0) -> (element=w200:cluster{"String":string, "Value":u16})
                n117 = Unbundle By Name(w200) -> ("Value"=w195:u16)
                n118 = property on="Parameter 5B" class="Ring (strict)"(error in=w197, "DisabledEnum"=w209, "Value"=w195) -> (error out=w196:errorcluster)  [unwired: 1 in, 1 out]
              }
              frame True {
                w222 = T4."Enabled" ("Disabled")
                n119 = Index Array(array=w234, index=1) -> (element=w233:string)
                n120 = property on="Parameter 1B" class="Ring (strict)"(error in=w221, "DisabledEnum"=w222) -> (error out=w236:errorcluster, "Strings []"=w237:string[])  [unwired: 1 in, 1 out]
                n121 = Search 1D Array(1D array=w237, element=w233) -> (index of element=w231:i32)  [unwired: 1 in]
                n122 = Increment(x=w231) -> (x+1=w220:i32)
                n123 = Index Array(array=w232, index=w220) -> (element=w230:T5)
                n124 = Unbundle By Name(w230) -> ("Event type"=w229:u16, "Time, s"=w228:sgl, "Stimulus, s"=w225:sgl, "TTL out"=w223:u16)
                n125 = property on="Parameter 1B" class="Ring (strict)"(error in=w236, "Value"=w231) -> (error out=w235:errorcluster)  [unwired: 1 in, 1 out]
                n126 = property on="Parameter 2B" class="Ring (strict)"(error in=w235, "Value"=w229, "DisabledEnum"=w222) -> (error out=w227:errorcluster)  [unwired: 1 in, 1 out]
                n127 = property on="Parameter 3B" class="DigNum (strict)"(error in=w227, "Value"=w228, "DisabledEnum"=w222) -> (error out=w226:errorcluster)  [unwired: 1 in, 1 out]
                n128 = property on="Parameter 4B" class="DigNum (strict)"(error in=w226, "Value"=w225, "DisabledEnum"=w222) -> (error out=w224:errorcluster)  [unwired: 1 in, 1 out]
                n129 = property on="Parameter 5B" class="Ring (strict)"(error in=w224, "Value"=w223, "DisabledEnum"=w222) -> (error out=w219:errorcluster)  [unwired: 1 in, 1 out]
              }
            }
            n130 = disable-structure shown="Disabled" {
              disable-tunnel: w162 -> [w194 _]
              disable-tunnel: w161 -> [w192 _]
              frame Disabled {
                n131 = invoke on="TTL firing conditions" class="Tree (strict)" method="Edit Tree Items.Sort Children"(error in=w194, "tag"=w192, "Sort Column"=0) -> ()  [unwired: 5 in, 8 out]
              }
              frame Enabled {
              }
            }
          }
        }
      }
      event "Save Settings": Value Change {
        n132 = event-data() -> ("OldVal"=w239:bool)  [unwired: 1 in, 5 out]
        n133 = property on="Save Settings" class="Bool (strict)"("Value"=w239) -> (error out=w242:errorcluster)  [unwired: 2 in, 1 out]
        n134 = flat-sequence {
          tunnel: w242 -> [w243]
          tunnel: [w243] -> w240
          tunnel: [w250] -> w241
          tunnel: w240 -> [w250]
          tunnel: w241 -> [w252]
          frame #0 {
            n135 = property on="Run time, s" class="DigNum (strict)"() -> ("Value"=→"Out Run time, s":dbl)  [unwired: 2 in, 2 out]
            n136 = property on="Run time pause, s" class="DigNum (strict)"() -> ("Value"=→"Out Run time stim, s":dbl)  [unwired: 2 in, 2 out]
            n137 = property on="Run time stim, s" class="DigNum (strict)"() -> ("Value"=→"Out Run time pause, s":dbl)  [unwired: 2 in, 2 out]
            n138 = property on="Run time threshold, s" class="DigNum (strict)"() -> ("Value"=→"Out Run time threshold, s":dbl)  [unwired: 2 in, 2 out]
            n139 = property on="Speed detection threshold, mm/s" class="DigNum (strict)"() -> ("Value"=→"Out Speed detection threshold, mm/s":dbl)  [unwired: 2 in, 2 out]
            n140 = property on="Zone-based stimulus presents" class="Arr (strict)"() -> ("Value"=→"Modified Zone-based stimulus presents":T1)  [unwired: 2 in, 2 out]
          }
          frame #1 {
            n141 = Wait (ms)(milliseconds to wait=u32 50) -> ()  [unwired: 1 out]
          }
          frame #2 {
            n142 = property on="Exit" class="Bool (strict)"(error in=w252, "Value"=TRUE ("Exit")) -> ()  [unwired: 1 in, 2 out]
          }
        }
      }
      event "Add Button": Value Change {
        n143 = event-data() -> ("OldVal"=w255:bool)  [unwired: 1 in, 5 out]
        n144 = property on="TTL firing conditions" class="Tree (strict)"() -> ("Value"=w256:string)  [unwired: 2 in, 2 out]
        n145 = invoke on="TTL firing conditions" class="Tree (strict)" method="Navigate Tree.Get Path"("tag"=w256) -> ("Navigate Tree:Get Path"=w257:string[])  [unwired: 3 in, 3 out]
        n146 = property on="Add Button" class="Bool (strict)"("Value"=w255) -> ()  [unwired: 2 in, 2 out]
        n147 = property on="Zone-based stimulus presents" class="Arr (strict)"() -> ("Value"=w254:T1)  [unwired: 2 in, 2 out]
        n148 = Index Array(array=w257, index=0) -> (element=w258:string)
        n149 = case shown="\"Running bouts TTL controls\"" w258 {
          tunnel: w257 -> [_ _]
          tunnel: w254 -> [_ w262]
          frame "Running bouts TTL controls" {
          }
          frame "Zones", Default {
            w278 = FALSE ("use system decimal point (T)")
            n150 = property on="Parameter 2B" class="Ring (strict)"() -> ("Strings []"=w274:string[])  [unwired: 2 in, 2 out]
            n151 = property on="Parameter 3B" class="DigNum (strict)"() -> ("Value"=w261:dbl)  [unwired: 2 in, 2 out]
            n152 = property on="Parameter 4B" class="DigNum (strict)"() -> ("Value"=w260:dbl)  [unwired: 2 in, 2 out]
            n153 = property on="Parameter 1B" class="Ring (strict)"() -> ("Value"=w272:u16, "Strings []"=w269:string[], "Disabled Items []"=w270:i32[])  [unwired: 2 in, 2 out]
            n154 = property on="Parameter 5B" class="Ring (strict)"() -> ("Strings []"=w276:string[], "Value"=w264:u16)  [unwired: 2 in, 2 out]
            n155 = Array Size(array=w269) -> (size(s)=w267:i32)
            n156 = Index Array(array=w269, index=w272) -> (element=w271:string)
            n157 = Build Array (concatenate)(w270, w272) -> (w265:i32[])
            n158 = Decrement(x=w264) -> (x-1=w263:u16)
            n159 = Array Size(array=w265) -> (size(s)=w268:i32)
            n160 = Index Array(array=w274, index=0) -> (element=w283:string)
            n161 = Number To Fractional String(use system decimal point (T)=w278, number=w261, precision (6)=i16 2) -> (F-format string=w281:string)  [unwired: 1 in]
            n162 = Number To Fractional String(use system decimal point (T)=w278, number=w260, precision (6)=i16 2) -> (F-format string=w277:string)  [unwired: 1 in]
            n163 = Index Array(array=w276, index=w263) -> (element=w275:string)
            n164 = Less Or Equal?(x=w268, y=w267) -> (x <= y?=w266:bool)
            n165 = Build Array(w283, w281, w277, w275) -> (w280:string[])
            n166 = case shown="True" w266 {
              tunnel: TRUE ("Child Only?") -> [_ w305]
              tunnel: w280 -> [_ w295]
              tunnel: w271 -> [_ w302]
              tunnel: w265 -> [_ w303]
              tunnel: w262 -> [_ w297]
              tunnel: w261 -> [_ w289]
              tunnel: w260 -> [_ w288]
              frame False {
              }
              frame True {
                w294 = TRUE ("Set/Clear")
                n167 = Bundle By Name(cluster=T5 {"Event type"=0, "Time, s"=0.0, "Stimulus, s"=0.0, "Set/Clear"=FALSE, "TTL out"=0, "Stim. has been set"=FALSE} ("Element to add"), "Event type"=u16 0, "Time, s"=w289, "Stimulus, s"=w288, "Set/Clear"=w294, "TTL out"=u16 1, "Stim. has been set"=w294) -> (w290:T5)
                n168 = call <vilib>:"Space Constant.vi"() -> ("String"=w301:string)
                n169 = property on="Parameter 1B" class="Ring (strict)"("Disabled Items []"=w303) -> (error out=w287:errorcluster)  [unwired: 2 in, 1 out]
                n170 = Search/Split String(string=w302, search string/char (-)=w301) -> (match + rest of string=w300:string)  [unwired: 1 in, 2 out]
                n171 = call <vilib>:"Trim Whitespace.vi"("string"=w300) -> ("trimmed string"=w299:string)  [unwired: 1 in]
                n172 = invoke on="TTL firing conditions" class="Tree (strict)" method="Edit Tree Items.Add Item"(error in=w287, "Parent Tag"="Zones", "Child Position"=-1, "Left Cell"=w302, "Child Text"=w295, "Child Only?"=w305) -> (error out=w286:errorcluster)  [unwired: 3 in, 8 out]
                n173 = Decimal String To Number(string=w299, default (0L)=u8 0) -> (number=w296:u8)  [unwired: 1 in, 1 out]
                n174 = Replace Array Subset(array=w297, new element=w290, index=w296) -> (w285:T1)
                n175 = property on="Zone-based stimulus presents" class="Arr (strict)"(error in=w286, "Val(Sgnl)"=w285) -> ()  [unwired: 1 in, 2 out]
              }
            }
          }
        }
      }
      event "Remove Button": Value Change {
        n176 = event-data() -> ("OldVal"=w309:bool)  [unwired: 1 in, 5 out]
        n177 = property on="TTL firing conditions" class="Tree (strict)"() -> ("Value"=w307:string)  [unwired: 2 in, 2 out]
        n178 = invoke on="TTL firing conditions" class="Tree (strict)" method="Navigate Tree.Get Path"("tag"=w307) -> ("Navigate Tree:Get Path"=w310:string[])  [unwired: 3 in, 3 out]
        n179 = property on="Remove Button" class="Bool (strict)"("Value"=w309) -> ()  [unwired: 2 in, 2 out]
        n180 = property on="Zone-based stimulus presents" class="Arr (strict)"() -> ("Value"=w308:T1)  [unwired: 2 in, 2 out]
        n181 = Index Array(array=w310, index=0) -> (element=w311:string)
        n182 = case shown="\"Running bouts TTL controls\"" w311 {
          selector: w311 -> [w321 _]
          tunnel: w310 -> [_ _]
          tunnel: w308 -> [_ w357]
          tunnel: w307 -> [w333 _]
          frame "Running bouts TTL controls" {
            w313 = 4.0 ("Run time threshold, s")
            w314 = 1.0 ("Run time stim, s")
            w315 = 5.0 ("Run time pause, s")
            w320 = 8.0 ("Parameter 5A")
            w340 = T4."Enabled" ("Disabled")
            n183 = property on="Parameter 1A" class="DigNum (strict)"("Value"=0.0 ("Parameter 1A"), "DisabledEnum"=w340) -> ()  [unwired: 2 in, 2 out]
            n184 = property on="Run time stim, s" class="DigNum (strict)"("Value"=w314) -> ()  [unwired: 2 in, 2 out]
            n185 = property on="Run time, s" class="DigNum (strict)"("Value"=0.0 ("Run time, s")) -> ()  [unwired: 2 in, 2 out]
            n186 = property on="Run time threshold, s" class="DigNum (strict)"("Value"=w313) -> ()  [unwired: 2 in, 2 out]
            n187 = property on="Run time pause, s" class="DigNum (strict)"("Value"=w315) -> ()  [unwired: 2 in, 2 out]
            n188 = property on="Speed detection threshold, mm/s" class="DigNum (strict)"("Value"=w320) -> ()  [unwired: 2 in, 2 out]
            n189 = property on="Parameter 2A" class="DigNum (strict)"("Value"=0.0 ("Parameter 2A"), "DisabledEnum"=w340) -> (error out=w342:errorcluster)  [unwired: 2 in, 1 out]
            n190 = property on="Parameter 3A" class="DigNum (strict)"(error in=w342, "Value"=0.0 ("Parameter 3A"), "DisabledEnum"=w340) -> (error out=w339:errorcluster)  [unwired: 1 in, 1 out]
            n191 = property on="Parameter 4A" class="DigNum (strict)"(error in=w339, "Value"=0.0 ("Parameter 4A"), "DisabledEnum"=w340) -> (error out=w341:errorcluster)  [unwired: 1 in, 1 out]
            n192 = property on="Parameter 5A" class="DigNum (strict)"(error in=w341, "Value"=w320, "DisabledEnum"=w340) -> (error out=w319:errorcluster)  [unwired: 1 in, 1 out]
            n193 = invoke on="TTL firing conditions" class="Tree (strict)" method="Edit Tree Items.Delete"(error in=w319, "tag"=w333) -> (error out=w322:errorcluster)  [unwired: 3 in, 4 out]
            n194 = Number To Fractional String(number=w315, precision (6)=i16 2) -> (F-format string=w327:string)  [unwired: 2 in]
            n195 = Number To Fractional String(number=w314, precision (6)=i16 2) -> (F-format string=w326:string)  [unwired: 2 in]
            n196 = Number To Fractional String(number=w313, precision (6)=i16 2) -> (F-format string=w325:string)  [unwired: 2 in]
            n197 = Number To Fractional String(number=w320, precision (6)=i16 2) -> (F-format string=w324:string)  [unwired: 2 in]
            n198 = Build Array(w327, w326, w325, w324) -> (w323:string[])
            n199 = invoke on="TTL firing conditions" class="Tree (strict)" method="Edit Tree Items.Add Item"(error in=w322, "Parent Tag"=w321, "Child Position"=-1, "Left Cell"="Detect N sec run. bouts" ("Left Cell String"), "Child Text"=w323) -> (error out=w318:errorcluster)  [unwired: 4 in, 8 out]
            n200 = property on="Update Zones" class="Bool (strict)"(error in=w318, "Val(Sgnl)"=TRUE ("Value (Signaling)")) -> ()  [unwired: 1 in, 2 out]
          }
          frame "Zones", Default {
            n201 = property on="Parameter 1B" class="Ring (strict)" props=["Value", "Strings []", "Disabled Items []", "StringsAndValues[]"]() -> ("Value"=w363:u16, "Strings []"=w362:string[], "Disabled Items []"=w353:i32[])  [unwired: 2 in, 3 out]
            n202 = Index Array(array=w362, index=w363) -> (element=w349:string)
            n203 = call <vilib>:"Space Constant.vi"() -> ("String"=w361:string)
            n204 = Search/Split String(string=w349, search string/char (-)=w361) -> (match + rest of string=w360:string)  [unwired: 1 in, 2 out]
            n205 = Index Array(array=w357, index=0) -> (element=w355:T5)
            n206 = call <vilib>:"Trim Whitespace.vi"("string"=w360) -> ("trimmed string"=w359:string)  [unwired: 1 in]
            n207 = Decimal String To Number(string=w359, default (0L)=u8 0) -> (number=w354:u8)  [unwired: 1 in, 1 out]
            n208 = Replace Array Subset(array=w357, new element=w355, index=w354) -> (w345:T1)
            n209 = Search 1D Array(1D array=w353, element=w354) -> (index of element=w352:i32)  [unwired: 1 in]
            n210 = Delete From Array(array=w353, length=w352, index=1) -> (array with subset deleted=w351:i32[])  [unwired: 1 out]
            n211 = property on="Parameter 1B" class="Ring (strict)"("Disabled Items []"=w351) -> (error out=w348:errorcluster)  [unwired: 2 in, 1 out]
            n212 = property on="TTL firing conditions" class="Tree (strict)"(error in=w348, "Value"="Zones" ("TTL firing conditions")) -> (error out=w346:errorcluster)  [unwired: 1 in, 1 out]
            n213 = invoke on="TTL firing conditions" class="Tree (strict)" method="Edit Tree Items.Delete"(error in=w346, "tag"=w349, "Delete Children"=FALSE ("Delete Children?")) -> (error out=w344:errorcluster)  [unwired: 2 in, 4 out]
            n214 = property on="Zone-based stimulus presents" class="Arr (strict)"(error in=w344, "Val(Sgnl)"=w345) -> ()  [unwired: 1 in, 2 out]
          }
        }
      }
      event "Modify Button": Value Change {
        n215 = event-data() -> ("OldVal"=w366:bool)  [unwired: 1 in, 5 out]
        n216 = property on="TTL firing conditions" class="Tree (strict)"() -> ("Value"=w365:string)  [unwired: 2 in, 2 out]
        n217 = invoke on="TTL firing conditions" class="Tree (strict)" method="Navigate Tree.Get Path"("tag"=w365) -> ("Navigate Tree:Get Path"=w367:string[])  [unwired: 3 in, 3 out]
        n218 = property on="Modify Button" class="Bool (strict)"("Value"=w366) -> ()  [unwired: 2 in, 2 out]
        n219 = property on="Zone-based stimulus presents" class="Arr (strict)"() -> ("Value"=w364:T1)  [unwired: 2 in, 2 out]
        n220 = Index Array(array=w367, index=0) -> (element=w368:string)
        n221 = case shown="\"Running bouts TTL controls\"" w368 {
          selector: w368 -> [w373 _]
          tunnel: w367 -> [_ _]
          tunnel: w365 -> [w379 w416]
          tunnel: w364 -> [_ w398]
          frame "Running bouts TTL controls" {
            n222 = property on="Parameter 1A" class="DigNum (strict)"() -> (error out=w382:errorcluster, "Value"=w378:dbl)  [unwired: 2 in, 1 out]
            n223 = property on="Run time, s" class="DigNum (strict)"("Value"=w378) -> ()  [unwired: 2 in, 2 out]
            n224 = property on="Parameter 2A" class="DigNum (strict)"(error in=w382) -> (error out=w397:errorcluster, "Value"=w377:dbl)  [unwired: 1 in, 1 out]
            n225 = property on="Run time pause, s" class="DigNum (strict)"("Value"=w377) -> ()  [unwired: 2 in, 2 out]
            n226 = Number To Fractional String(number=w377, precision (6)=i16 2) -> (F-format string=w388:string)  [unwired: 2 in]
            n227 = property on="Parameter 3A" class="DigNum (strict)"(error in=w397) -> (error out=w395:errorcluster, "Value"=w376:dbl)  [unwired: 1 in, 1 out]
            n228 = property on="Parameter 4A" class="DigNum (strict)"(error in=w395) -> (error out=w396:errorcluster, "Value"=w375:dbl)  [unwired: 1 in, 1 out]
            n229 = property on="Run time threshold, s" class="DigNum (strict)"("Value"=w375) -> ()  [unwired: 2 in, 2 out]
            n230 = property on="Parameter 5A" class="DigNum (strict)"(error in=w396) -> (error out=w381:errorcluster, "Value"=w374:dbl)  [unwired: 1 in, 1 out]
            n231 = invoke on="TTL firing conditions" class="Tree (strict)" method="Edit Tree Items.Delete"(error in=w381, "tag"=w379) -> (error out=w383:errorcluster)  [unwired: 3 in, 4 out]
            n232 = property on="Speed detection threshold, mm/s" class="DigNum (strict)"("Value"=w374) -> ()  [unwired: 2 in, 2 out]
            n233 = Number To Fractional String(number=w376, precision (6)=i16 2) -> (F-format string=w387:string)  [unwired: 2 in]
            n234 = Number To Fractional String(number=w375, precision (6)=i16 2) -> (F-format string=w386:string)  [unwired: 2 in]
            n235 = Number To Fractional String(number=w374, precision (6)=i16 2) -> (F-format string=w385:string)  [unwired: 2 in]
            n236 = Build Array(w388, w387, w386, w385) -> (w384:string[])
            n237 = invoke on="TTL firing conditions" class="Tree (strict)" method="Edit Tree Items.Add Item"(error in=w383, "Parent Tag"=w373, "Child Position"=-1, "Left Cell"="Detect N sec run. bouts" ("Left Cell String"), "Child Text"=w384, "Child Only?"=TRUE) -> (error out=w372:errorcluster)  [unwired: 3 in, 8 out]
            n238 = property on="TTL firing conditions" class="Tree (strict)"(error in=w372, "Value"=w373) -> (error out=w371:errorcluster)  [unwired: 1 in, 1 out]
            n239 = property on="Update Zones" class="Bool (strict)"(error in=w371, "Val(Sgnl)"=TRUE ("Value (Signaling)")) -> ()  [unwired: 1 in, 2 out]
            n240 = property on="Run time stim, s" class="DigNum (strict)"("Value"=w376) -> ()  [unwired: 2 in, 2 out]
          }
          frame "Zones", Default {
            w408 = TRUE ("Set/Clear")
            w429 = FALSE ("use system decimal point (T)")
            n241 = property on="Parameter 1B" class="Ring (strict)"() -> ("Value"=w423:u16, "Strings []"=w422:string[])  [unwired: 2 in, 2 out]
            n242 = property on="Parameter 2B" class="Ring (strict)"() -> ("Strings []"=w425:string[])  [unwired: 2 in, 2 out]
            n243 = property on="Parameter 3B" class="DigNum (strict)"() -> ("Value"=w400:dbl)  [unwired: 2 in, 2 out]
            n244 = property on="Parameter 4B" class="DigNum (strict)"() -> ("Value"=w399:dbl)  [unwired: 2 in, 2 out]
            n245 = property on="Parameter 5B" class="Ring (strict)"() -> ("Strings []"=w427:string[], "Value"=w415:u16)  [unwired: 2 in, 2 out]
            n246 = Bundle By Name(cluster=T5 {"Event type"=0, "Time, s"=0.0, "Stimulus, s"=0.0, "Set/Clear"=FALSE, "TTL out"=0, "Stim. has been set"=FALSE} ("Element to add"), "Event type"=u16 0, "Time, s"=w400, "Stimulus, s"=w399, "Set/Clear"=w408, "TTL out"=u16 1, "Stim. has been set"=w408) -> (w412:T5)
            n247 = Index Array(array=w422, index=w423) -> (element=w401:string)
            n248 = Decrement(x=w415) -> (x-1=w414:u16)
            n249 = call <vilib>:"Space Constant.vi"() -> ("String"=w403:string)
            n250 = Index Array(array=w425, index=0) -> (element=w434:string)
            n251 = Number To Fractional String(use system decimal point (T)=w429, number=w400, precision (6)=i16 3) -> (F-format string=w432:string)  [unwired: 1 in]
            n252 = Number To Fractional String(use system decimal point (T)=w429, number=w399, precision (6)=i16 3) -> (F-format string=w428:string)  [unwired: 1 in]
            n253 = Index Array(array=w427, index=w414) -> (element=w426:string)
            n254 = Search/Split String(string=w401, search string/char (-)=w403) -> (match + rest of string=w404:string)  [unwired: 1 in, 2 out]
            n255 = Build Array(w434, w432, w428, w426) -> (w431:string[])
            n256 = call <vilib>:"Trim Whitespace.vi"("string"=w404) -> ("trimmed string"=w405:string)  [unwired: 1 in]
            n257 = Decimal String To Number(string=w405, default (0L)=u8 0) -> (number=w407:u8)  [unwired: 1 in, 1 out]
            n258 = Replace Array Subset(array=w398, new element=w412, index=w407) -> (w413:T1)
            n259 = invoke on="TTL firing conditions" class="Tree (strict)" method="Edit Tree Items.Delete"("tag"=w416) -> (error out=w417:errorcluster)  [unwired: 4 in, 4 out]
            n260 = property on="Update Zones" class="Bool (strict)"("Val(Sgnl)"=TRUE ("Value (Signaling)")) -> ()  [unwired: 2 in, 2 out]
            n261 = invoke on="TTL firing conditions" class="Tree (strict)" method="Edit Tree Items.Add Item"(error in=w417, "Parent Tag"="Zones", "Child Position"=-1, "Left Cell"=w401, "Child Text"=w431, "Child Only?"=TRUE) -> (error out=w402:errorcluster)  [unwired: 3 in, 8 out]
            n262 = property on="Zone-based stimulus presents" class="Arr (strict)"(error in=w402, "Val(Sgnl)"=w413) -> ()  [unwired: 1 in, 2 out]
          }
        }
      }
      event Timeout {
        n263 = event-data() -> ()  [unwired: 1 in, 3 out]
      }
      event "Zone-based stimulus presents": Value Change {
        n264 = event-data() -> ("OldVal"=→"OldVal":T1, "NewVal"=→"NewVal":T1)  [unwired: 1 in, 4 out]
        n265 = property on="Update Zones" class="Bool (strict)"("Val(Sgnl)"=TRUE ("Value (Signaling)")) -> ()  [unwired: 2 in, 2 out]
      }
    }
  }
